vi "RPC Method PerformOCVMeasurement.vi"(8 "error in (no error)":errorcluster, 11 "OOP Server in":refnum<class "OCV4.lvclass">) -> (0 "error out":errorcluster, 3 "OOP Server out":refnum<class "OCV4.lvclass">)   [LabVIEW 2019, in "OCV4.lvlib" / "OCV4.lvclass"]
uses:
  OCV4.lvclass
  OCV4.lvclass/OCV4.ctl
  RPC Messages/measurementservice_ErrorOut/measurementservice_ErrorOut_Data.ctl
  RPC Messages/measurementservice_OCVRaw/measurementservice_OCVRaw_Data.ctl
  RPC Messages/measurementservice_OCVData/measurementservice_OCVData_Data.ctl
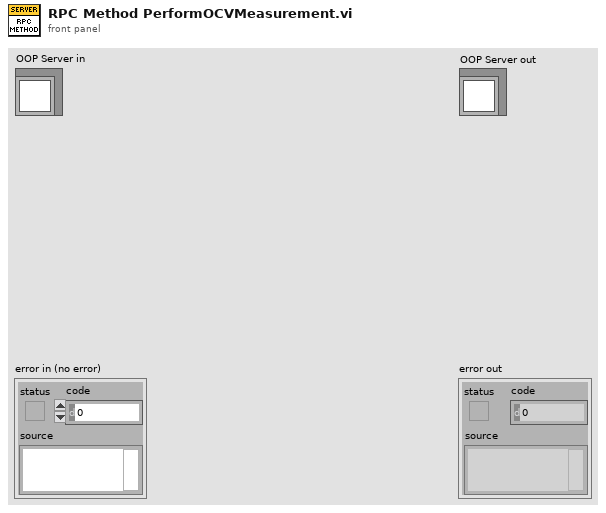
[diagram p1: front panel]
types:
  T1 = typedef "OCV4.lvlib/OCV4.lvclass/measurementservice_ErrorOut_Data.ctl" = cluster{"errCode":i32, "errMessage":string}
  T2 = typedef "OCV4.lvlib/OCV4.lvclass/measurementservice_OCVRaw_Data.ctl" = cluster{"battery1voltage":sgl, "battery2voltage":sgl, "battery3voltage":sgl, "error":T1}
  T3 = typedef "OCV4.lvlib/OCV4.lvclass/measurementservice_OCVData_Data.ctl" = cluster{"data":T2[]}
  T4 = typedef "OCV4.lvlib/OCV4.lvclass/Server Internal UEs.ctl" = cluster{"Invoke Internal UE":refnum<user-event>, "Query Internal UE":refnum<user-event>, "PerformOCVMeasurement Internal UE":refnum<user-event>, "PerformACIRMeasurement Internal UE":refnum<user-event>, "StreamOCVMeasurement Internal UE":refnum<user-event>, "Register Internal UE":refnum<user-event>}
  T5 = typedef "OCV4.lvlib/OCV4.lvclass/Server gRPC UEs.ctl" = cluster{"Invoke gRPC UE":refnum<user-event>, "Query gRPC UE":refnum<user-event>, "PerformOCVMeasurement gRPC UE":refnum<user-event>, "PerformACIRMeasurement gRPC UE":refnum<user-event>, "StreamOCVMeasurement gRPC UE":refnum<user-event>, "Register gRPC UE":refnum<user-event>}
  T6 = typedef "OCV4.lvlib/gprc-lvsupport.lvlib/grpcId.ctl" = u64
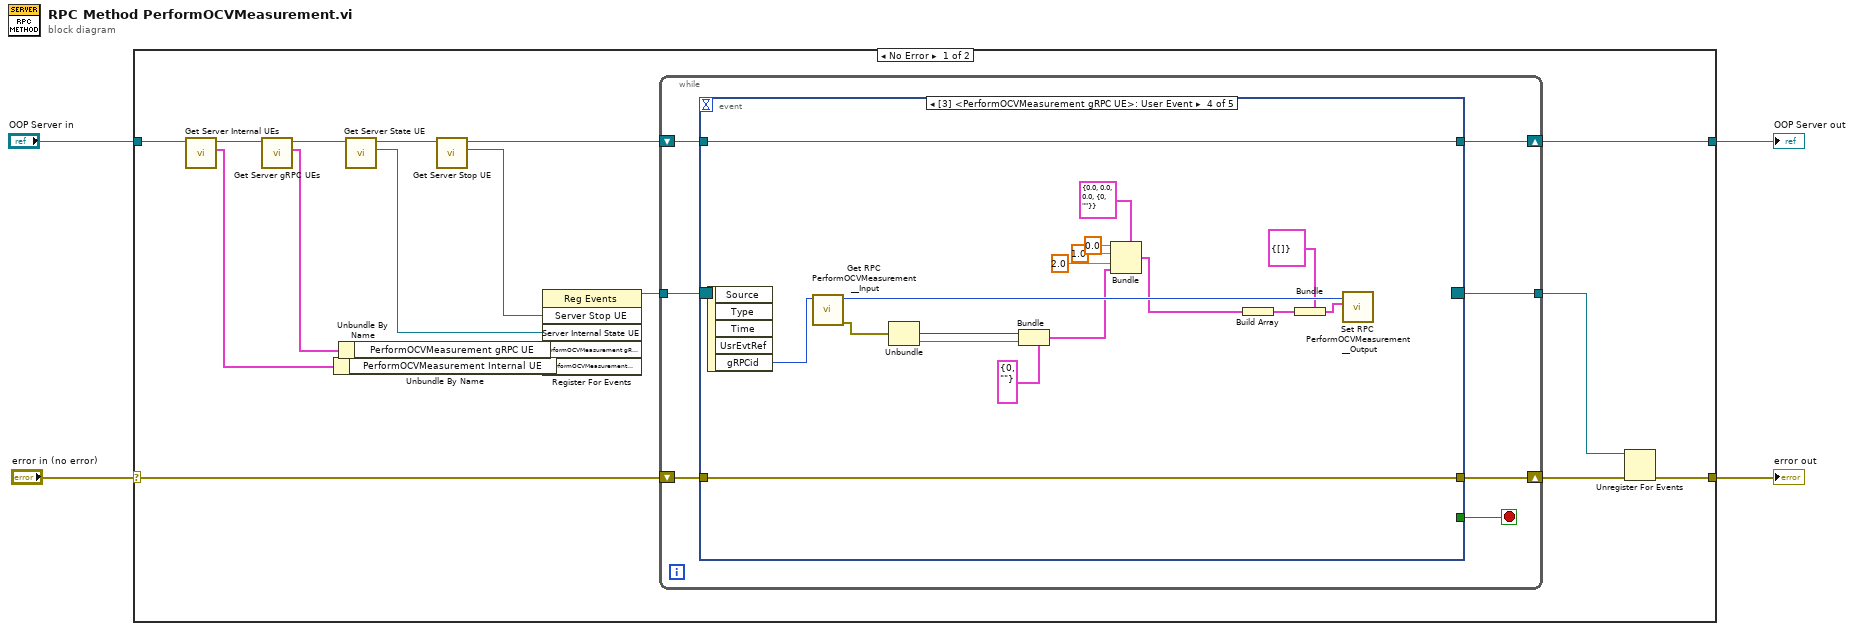
[diagram p0: block diagram]
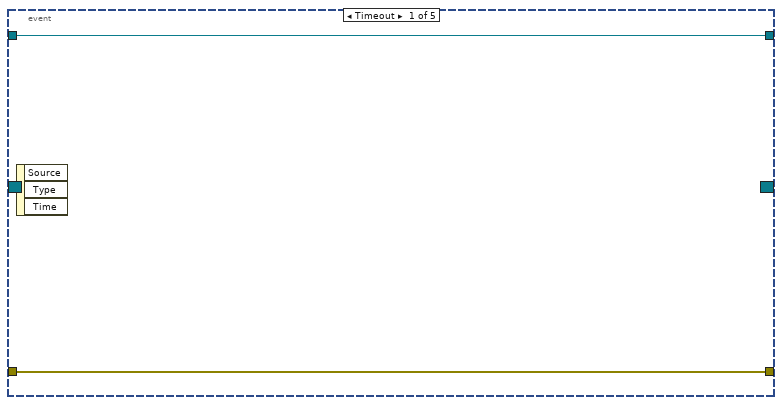
[diagram p2: hidden frame]
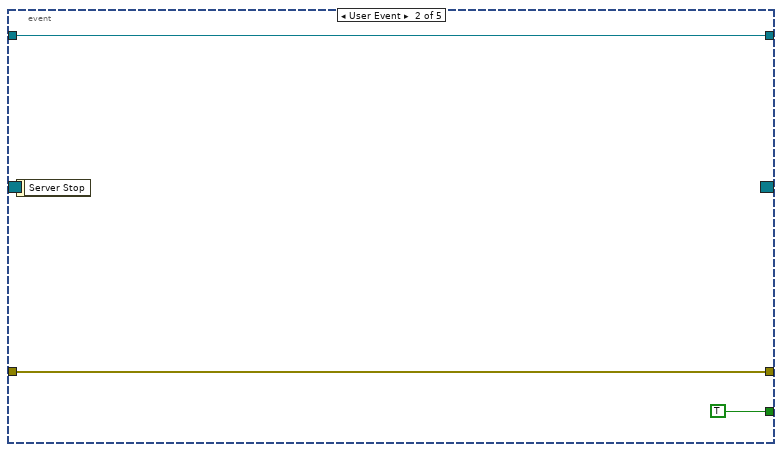
[diagram p3: hidden frame]
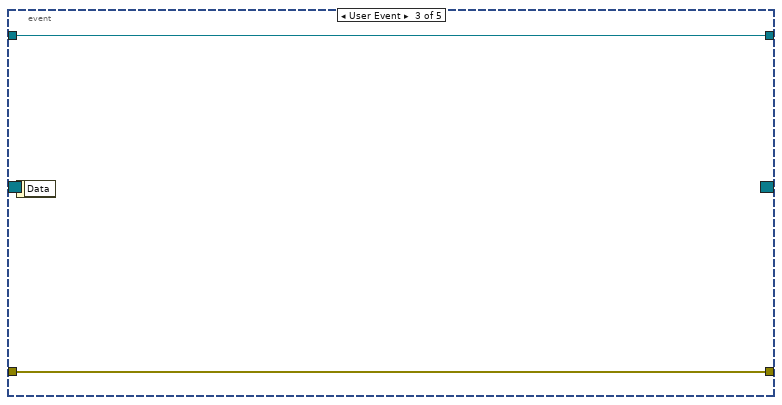
[diagram p4: hidden frame]
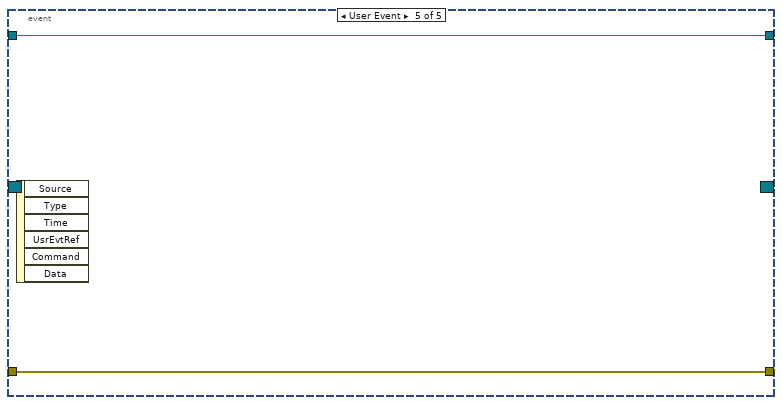
[diagram p5: hidden frame]
diagram:
  n1 = case shown="No Error" "error in (no error)" {
    selector: "error in (no error)" -> [w17 w56]
    tunnel: [w15 w56] -> w3
    tunnel: "OOP Server in" -> [w19 w55]
    tunnel: [w5 w55] -> w1
    frame No Error {
      n2 = call "Get Server Internal UEs.vi"("OOP Server in"=w19) -> ("Server Internal UEs"=w11:T4, "OOP Server out"=w18:refnum<class "OCV4.lvclass">)  [unwired: 9 in]
      n3 = call "Get Server gRPC UEs.vi"("OOP Server in"=w18) -> ("Server gRPC UEs"=w13:T5, "OOP Server out"=w8:refnum<class "OCV4.lvclass">)  [unwired: 9 in]
      n4 = Unbundle By Name ("Unbundle Internal UE")(w11) -> ("PerformOCVMeasurement Internal UE"=w10:refnum<user-event>)
      n5 = Unbundle By Name ("Unbundle gRPC UE")(w13) -> ("PerformOCVMeasurement gRPC UE"=w12:refnum<user-event>)
      n6 = call "Get Server State UE.vi"("Template Server in"=w8) -> ("Server Internal State UE"=w6:refnum<user-event>, "Template Server out"=w7:refnum<class "OCV4.lvclass">)  [unwired: 9 in]
      n7 = call "Get Server Stop UE.vi"("OOP Server in"=w7) -> ("Server Stop UE"=w21:refnum<user-event>, "OOP Server out"=w9:refnum<class "OCV4.lvclass">)  [unwired: 9 in]
      n8 = register-events(w21, w6, w12, w10) -> (reference out=w20:refnum<event-registration>)  [unwired: 2 in, 1 out]
      n9 = while {
        tunnel: w20 -> [w28]
        tunnel: [w24] -> w14
        shift-right: [w25] -> w16
        shift-left: w17 -> [w26]
        shift-right: [w22] -> w5
        shift-left: w9 -> [w23]
        stop <- w27 stop-if-true
        n10 = event "RPC Method Event Structure" shown="[3] <PerformOCVMeasurement gRPC UE>: User Event" {
          selector: w28 -> [_ _ _ _ _]
          dyn-events: [_ _ _ _ _] -> w24
          timeout: _ -> [_ _ _ _ _]
          tunnel: [_ TRUE _ _ _] -> w27
          tunnel: w26 -> [w30 w32 w35 w52 w54]
          tunnel: [w30 w32 w35 w52 w54] -> w25
          tunnel: w23 -> [w29 w31 w34 w51 w53]
          tunnel: [w29 w31 w34 w51 w53] -> w22
          event Timeout {
            n11 = event-data() -> ()  [unwired: 1 in, 3 out]
          }
          event User Event {
            n12 = event-data() -> ()  [unwired: 1 in, 1 out]
          }
          event User Event {
            n13 = event-data() -> ()  [unwired: 1 in, 1 out]
          }
          event User Event {
            n14 = event-data() -> ("gRPCid"=w50:T6)  [unwired: 1 in, 4 out]
            n15 = call "Get RPC PerformOCVMeasurement __Input.vi"("gRPCid in"=w50) -> ("error out"=w40:errorcluster, "gRPCid out"=w49:T6)  [unwired: 8 in, 1 out]
            n16 = Unbundle(w40) -> ("code"=w38:i32, "source"=w37:string)  [unwired: 1 out]
            n17 = Bundle(cluster=T1 {"errCode"=0, "errMessage"=""} ("measurementservice_ErrorOut_Data"), "errCode"=w38, "errMessage"=w37) -> (w36:T1)
            n18 = Bundle(cluster=T2 {"battery1voltage"=0.0, "battery2voltage"=0.0, "battery3voltage"=0.0, "error"={"errCode"=0, "errMessage"=""}} ("measurementservice_OCVRaw_Data"), "battery1voltage"=sgl 0.0, "battery2voltage"=sgl 1.0, "battery3voltage"=sgl 2.0, "error"=w36) -> (w45:T2)
            n19 = Build Array(w45) -> (w44:T2[])
            n20 = Bundle(cluster=T3 {"data"=[]} ("Message Data"), "data"=w44) -> (w47:T3)
            n21 = call "Set RPC PerformOCVMeasurement __Output.vi"("Message Data"=w47, "gRPCid in"=w49) -> ()  [unwired: 9 in, 1 out]
          }
          event User Event {
            n22 = event-data() -> ()  [unwired: 1 in, 6 out]
          }
        }
      }
      n23 = Unregister For Events(event registration refnum=w14, error in=w16) -> (error out=w15:errorcluster)
    }
    frame Error {
    }
  }
  "error out" <- w3
  "OOP Server out" <- w1
